vi "LVClass_HasoSlopes Get Info.vi"(0 "HasoSlopes in":refnum<class "HasoSlopes.lvclass">, 11 "error in (no error)":errorcluster) -> (4 "HasoSlopes out":refnum<class "HasoSlopes.lvclass">, 8 "dimension":cluster{"size":T1, "step":T2}, 10 "HASO serial number":string, 14 "current time":timestamp, 15 "error out":errorcluster)   [LabVIEW 2020, in "HasoSlopes.lvclass"]
doc: "HasoSlopes specifications getter.\n\n--------------------------------------------------------------------------------\n\n<B>HasoSlopesIn </B> : HasoSlopes object.\n<B>HasoSlopesOut </B> : HasoSlopes object.\n<B>serial_number </B> : Serial number.\n<B>dimensions </B> : Pupil dimensions (width, height)\n<B>steps </B> : Subpupil size (um).\n<B>ErrorIn </B> : Error\n<B>ErrorOut </B> : Error\n\n--------------------------------------------------------------------------------"
uses:
  HasoSlopes.lvclass
  Controls/Point2D.ctl
  Controls/Point2Df.ctl
  HasoSlopes.lvclass/HasoSlopes.ctl
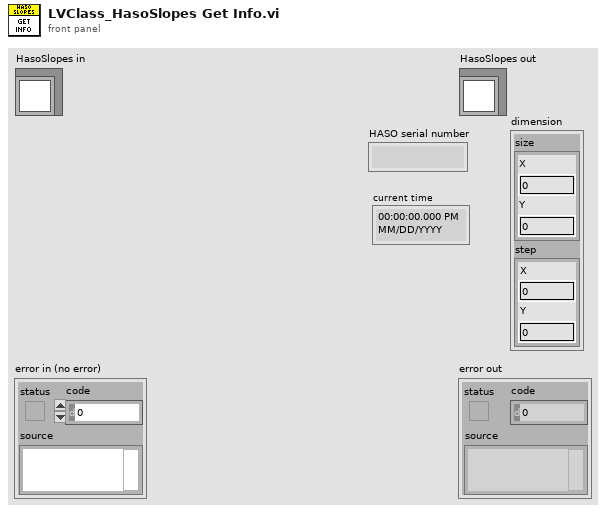
[diagram p1: front panel]
types:
  T1 = typedef "Point2D.ctl" = cluster{"X":u32, "Y":u32}
  T2 = typedef "Point2Df.ctl" = cluster{"X":sgl, "Y":sgl}
  T3 = typedef "ClassID.ctl" = i64
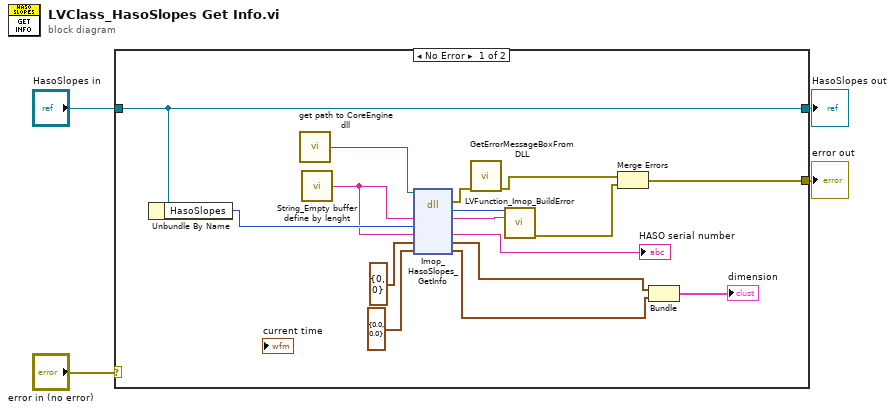
[diagram p0: block diagram]
diagram:
  n1 = case shown="No Error" "error in (no error)" {
    selector: "error in (no error)" -> [_ w22]
    tunnel: [w5 w22] -> w3
    tunnel: [w18 w21] -> w1
    tunnel: "HasoSlopes in" -> [w18 w21]
    frame No Error {
      n2 = Unbundle By Name(w18) -> ("HasoSlopes"=w17:T3)
      n3 = call "get path to CoreEngine dll.vi"() -> ("path to wavekit library"=w16:path)  [unwired: 14 in, 1 out]
      n4 = call "String_Empty buffer define by lenght.vi"() -> ("Empty buffer"=w11:string)  [unwired: 1 in]
      n5 = dll-call lib="D:/2_trunk/Soft_haso/ImOpCoreEngine4_LV2011/DLLs/ImopEngine4_vc100.dll" fn="Imop_HasoSlopes_GetInfo"(path in=w16, "message"=w11, "objet"=w17, "numserie"=w11, "size"=T1 {"X"=0, "Y"=0} ("Size1"), "step"=T2 {"X"=0.0, "Y"=0.0} ("Step")) -> (error out=w15:errorcluster, "return type"=w19:i32, "message"=w20:string, "numserie"=→"HASO serial number":string, "size"=w10:T1, "step"=w9:T2)  [unwired: 3 in, 1 out]
      n6 = call "GetErrorMessageBoxFromDLL.vi"("error IN"=w15) -> ("error OUT"=w7:errorcluster)  [unwired: 10 in]
      n7 = call "LVFunction_Imop_BuildError.vi"("code"=w19, "String to Prepend to source (\"\")"=w20) -> ("error out"=w6:errorcluster)  [unwired: 13 in]
      n8 = Merge Errors(w7, w6) -> (w5:errorcluster)
      n9 = Bundle("size"=w10, "step"=w9) -> (→"dimension":cluster{"size":T1, "step":T2})  [unwired: 1 in]
    }
    frame Error {
    }
  }
  "error out" <- w3
  "HasoSlopes out" <- w1
